vi "BRig_dataBlock_c_nReward_total_L.vi"() -> (2 "output_nReward_total_L":i32)   [LabVIEW 2014]
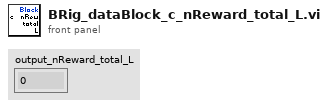
[diagram p1: front panel]
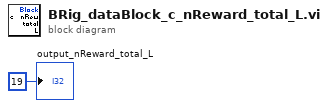
[diagram p0: block diagram]
diagram:
  "output_nReward_total_L" <- 19 ("output_iBlock")
